vi "Main.vi"(11 "Module Admin":refnum<class "Delacor_lib_QMH_Module Admin.lvclass">) -> ()   [LabVIEW 2024, in "Settings Editor.lvlib"]
doc: "This template is based off of the Queued Message Handler design pattern and the Queued Message Handler project template that ships with LabVIEW.\n\nThe main difference is that the queue is private to this module and communication between modules is performed via Broadcast and Request events.\n\nRequest events are wrapped in public API methods and are handled in the Event Handling Loop (EHL) of this VI. Any module can register for Broadcast events sent by this module. The EHL generates messages based on user interface actions.\n\nThe Message Handling Loop (MHL) processes messages generated by the EHL, or by other messages. The messages are string values, so new messages can be added easily to the Message Cases case structure in the MHL. Each message cluster can also provide an optional value for Message Data, which is a variant that can be converted to whatever message-specific data is required.\n_____\nBased on DQMH Project Template 4.0.0.47.\n_____\nBased on DQMH Dev Tools: Project Template 7.1.0.1503."
uses:
  Settings Editor.lvlib
  <vilib>/Delacor/Delacor QMH/Libraries/Module Admin_class/Delacor_lib_QMH_Module Admin.lvclass
  CML Shared/Signal Type--enum.ctl
  CML Shared/Calibration Values--cluster.ctl
  Module Data--cluster.ctl
  Settings--cluster.ctl
  <vilib>/Delacor/Delacor QMH/Libraries/Message Queue_class/Delacor_lib_QMH_Message Queue.lvclass/Delacor_lib_QMH_Message Queue.ctl
  Stop Argument--cluster.ctl
  Update Application Settings Argument--cluster.ctl
  Update Application Settings (Reply Payload)--cluster.ctl
  <vilib>/Delacor/Delacor QMH/Libraries/Module Admin_class/Delacor_lib_QMH_Module Admin.lvclass/Delacor_lib_QMH_Module Admin.ctl
  <vilib>/Utility/miscctls.llb/LVPointTypeDef.ctl
  <vilib>/Delacor/Delacor QMH/Libraries/Message Queue_class/Delacor_lib_QMH_Enqueue Message (Single).vi
  <vilib>/Delacor/Delacor QMH/Libraries/Module Admin_class/Delacor_lib_QMH_Get External Launch.vi
  <vilib>/Delacor/Delacor QMH/Libraries/Message Queue_class/Delacor_lib_QMH_Message Queue.lvclass
  CML Shared/CML Shared.lvlib
panel:
  in  "Open API TESTERS Window for Debug":bool
  in  "Calibration Values":T1[](array[typedef])
  in  "Cancel":bool
  in  "OK":bool
  in  "Log File Base Path":path
  in  "Signal Type":T2
  out "error out":errorcluster
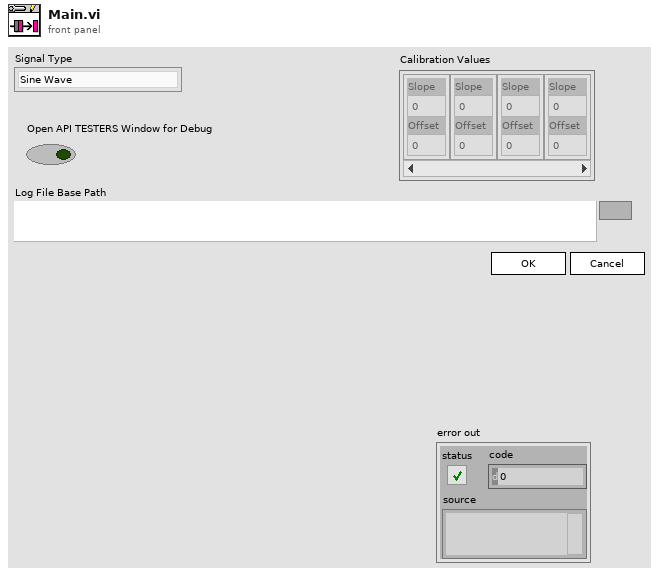
[diagram p1: front panel]
types:
  T1 = typedef "CML Shared.lvlib/Calibration Values--cluster.ctl" = cluster{"Slope":dbl, "Offset":dbl}
  T2 = typedef "CML Shared.lvlib/Signal Type--enum.ctl" = enum16{"Sine Wave", "Square with Noise"}
  T3 = typedef "Settings Editor.lvlib/Request Events--cluster.ctl" = cluster{"Stop Module":refnum<user-event>, "Show Panel":refnum<user-event>, "Hide Panel":refnum<user-event>, "Get Module Execution Status":refnum<user-event>, "Show Diagram":refnum<user-event>, "Update Application Settings":refnum<user-event>}
  T4 = typedef "Settings Editor.lvlib/Module Data--cluster.ctl" = cluster{"Settings":T5}
  T5 = typedef "Settings Editor.lvlib/Settings--cluster.ctl" = cluster{"Signal Type":T2, "Calibration Array":T1[], "Log File Base Path":path}
  T6 = enum32{"invalid lock state", "Not Locked", "Locked (No Password)", "Password-protected"}
  T7 = typedef "Settings Editor.lvlib/Stop Argument--cluster.ctl" = cluster{"Origin":string, "Exit via Stop Module Req?":bool, "Wait for Module to stop?":bool}
  T8 = typedef "Settings Editor.lvlib/Update Application Settings Argument--cluster.ctl" = cluster{"Wait Notifier":refnum<notifier>, "wait for reply":bool}
  T9 = typedef "LVPointTypeDef.ctl" = cluster{"Horizontal":i16, "Vertical":i16}
  T10 = enum32{"Invalid", "Standard", "Closed", "Hidden", "Minimized", "Maximized"}
  T11 = typedef "Settings Editor.lvlib/Update Application Settings (Reply Payload)--cluster.ctl" = cluster{"Settings":T5, "error":errorcluster}
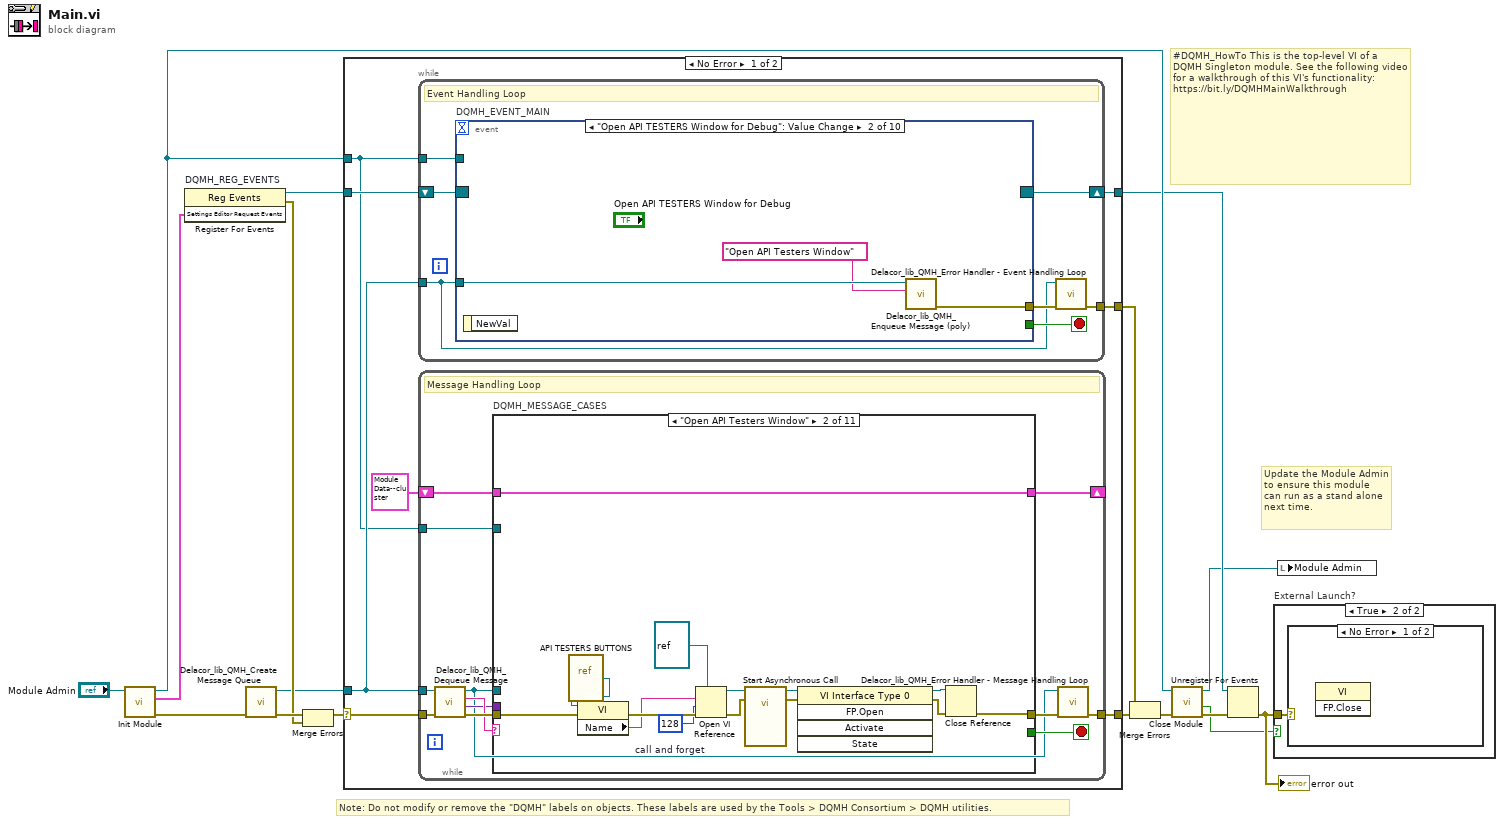
[diagram p0: block diagram]
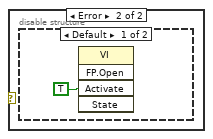
[diagram p3: hidden frame]
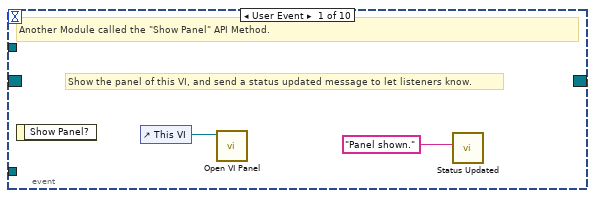
[diagram p5: hidden frame]
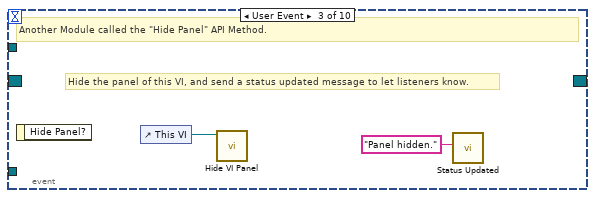
[diagram p6: hidden frame]
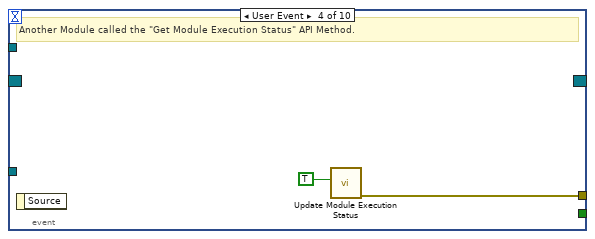
[diagram p7: hidden frame]
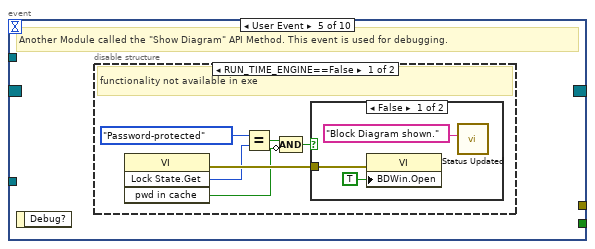
[diagram p8: hidden frame]
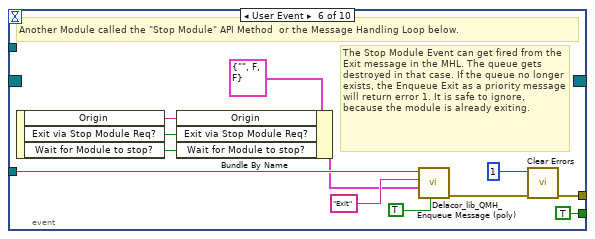
[diagram p11: hidden frame]
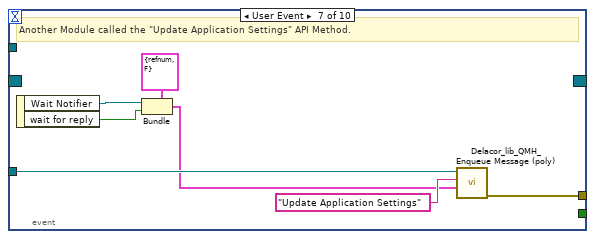
[diagram p12: hidden frame]
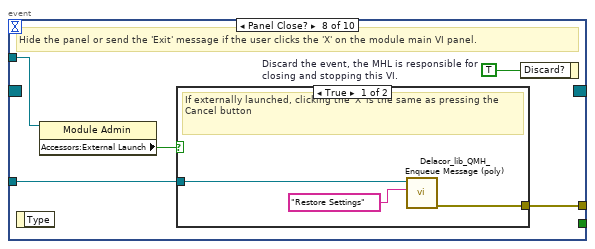
[diagram p13: hidden frame]
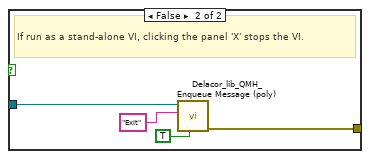
[diagram p14: hidden frame]
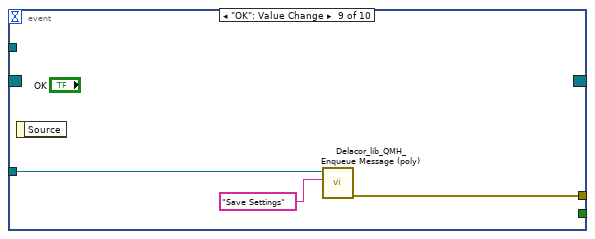
[diagram p15: hidden frame]
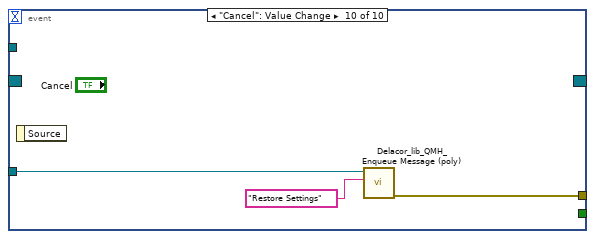
[diagram p16: hidden frame]
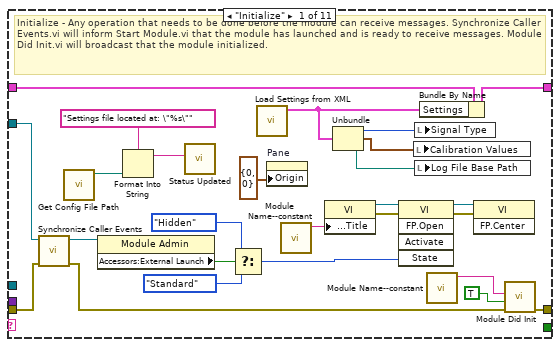
[diagram p17: hidden frame]
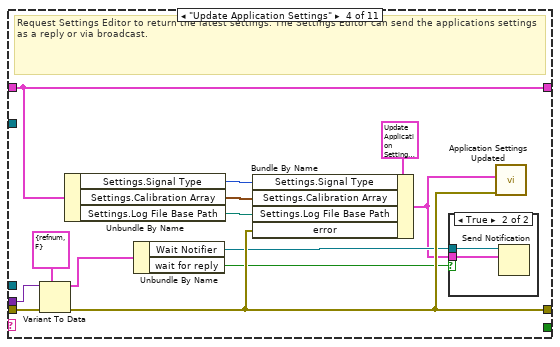
[diagram p19: hidden frame]
diagram:
  # "#DQMH_HowTo This is the top-level VI of a DQMH Singleton module. See the following video for a walkthrough of this VI's functionality: https://bit.ly/DQMHMainWalkthrough"
  # "Note: Do not modify or remove the \"DQMH\" labels on objects. These labels are used by the Tools > DQMH Consortium > DQMH utilities."
  # "Update the Module Admin to ensure this module can run as a stand alone next time."
  n1 = call "Init Module.vi"("Singleton Module Admin in"="Module Admin") -> ("error out"=w16:errorcluster, "Settings Editor Request Events"=w5:T3, "Singleton Module Admin out"=w8:refnum<class "Delacor_lib_QMH_Module Admin.lvclass">)  [unwired: 8 in]
  n2 = register-events "DQMH_REG_EVENTS"(w5) -> (reference out=w6:refnum<event-registration>, error out=w9:errorcluster)  [unwired: 2 in]
  n3 = call <vilib>:"Delacor_lib_QMH_Create Message Queue.vi"("error in"=w16) -> ("error out"=w11:errorcluster, "Message Queue"=w4:refnum<class "Delacor_lib_QMH_Message Queue.lvclass">)  [unwired: 9 in]
  n4 = Merge Errors(w11, w9) -> (w10:errorcluster)
  n5 = case shown="No Error" w10 {
    selector: w10 -> [w23 w230]
    tunnel: [w25 w229] -> w17
    tunnel: [w22 w228] -> w7
    tunnel: w6 -> [w20 w228]
    tunnel: w4 -> [w19 w223]
    tunnel: [w24 _] -> w14
    tunnel: w8 -> [w18 w224]
    frame No Error {
      n6 = while {
        tunnel: w19 -> [w26]
        shift-right: [w29] -> w22
        shift-left: w20 -> [w30]
        tunnel: [w31] -> w24
        tunnel: w18 -> [w27]
        stop <- w28 stop-if-true
        # "Event Handling Loop"
        n7 = event "DQMH_EVENT_MAIN" shown="[1] \"Open API TESTERS Window for Debug\": Value Change" {
          selector: w30 -> [_ _ _ _ _ _ _ _ _ _]
          dyn-events: [_ _ _ _ _ _ _ _ _ _] -> w29
          timeout: _ -> [_ _ _ _ _ _ _ _ _ _]
          tunnel: [_ _ _ _ _ TRUE ("Discard?") _ _ _ _] -> w28
          tunnel: w26 -> [_ w36 _ _ _ w58 w68 w72 w82 w85]
          tunnel: [_ w37 _ w41 _ w61 w69 w74 w84 w87] -> w32
          tunnel: w27 -> [_ _ _ _ _ _ _ w71 _ _]
          event User Event {
            # "Show the panel of this VI, and send a status updated message to let listeners know."
            # "Another Module called the \"Show Panel\" API Method."
            n8 = event-data() -> ()  [unwired: 1 in, 1 out]
            n9 = control-ref of="This VI"() -> (w34:refnum<vi>)
            n10 = call "Open VI Panel.vi"("VI"=w34) -> ()  [unwired: 10 in, 1 out]
            n11 = call "Status Updated.vi"("Status"="Panel shown." ("format string")) -> ()  [unwired: 10 in, 1 out]
          }
          event "Open API TESTERS Window for Debug": Value Change {
            n12 = event-data() -> ()  [unwired: 1 in, 1 out]
            n13 = call-poly <vilib>:"Delacor_lib_QMH_Enqueue Message (poly).vi"("Message"="Open API Testers Window", "Message Queue in"=w36) -> ("error out"=w37:errorcluster)  [unwired: 8 in, 1 out]
          }
          event User Event {
            # "Hide the panel of this VI, and send a status updated message to let listeners know."
            # "Another Module called the \"Hide Panel\" API Method."
            n14 = event-data() -> ()  [unwired: 1 in, 1 out]
            n15 = control-ref of="This VI"() -> (w39:refnum<vi>)
            n16 = call "Hide VI Panel.vi"("VI"=w39) -> ()  [unwired: 10 in, 1 out]
            n17 = call "Status Updated.vi"("Status"="Panel hidden." ("format string")) -> ()  [unwired: 10 in, 1 out]
          }
          event User Event {
            # "Another Module called the \"Get Module Execution Status\" API Method."
            n18 = event-data() -> ()  [unwired: 1 in, 1 out]
            n19 = call "Update Module Execution Status.vi"("Running?"=TRUE) -> ("error out"=w41:errorcluster)  [unwired: 10 in]
          }
          event User Event {
            # "Another Module called the \"Show Diagram\" API Method. This event is used for debugging."
            n20 = event-data() -> ()  [unwired: 1 in, 1 out]
            n21 = disable-structure shown="RUN_TIME_ENGINE==False" {
              frame condition #0 (active) {
                # "functionality not available in exe"
                n22 = invoke on="Invoke Node" class="VI" method="Lock State.Get"() -> (error out=w47:errorcluster, "Get Lock State"=w46:T6, "pwd in cache"=w43:bool)  [unwired: 4 in, 1 out]
                n23 = Equal?(x=T6."Password-protected", y=w46) -> (x = y?=w44:bool)
                n24 = Compound Arithmetic op=AND(w44, invert w43) -> (w42:bool)
                n25 = case shown="False" w42 {
                  tunnel: w47 -> [w50 _]
                  frame False {
                    n26 = property on="Property Node" class="VI"(error in=w50, "BDWin.Open"=TRUE ("Block Diagram Window:Open")) -> ()  [unwired: 1 in, 2 out]
                    n27 = call "Status Updated.vi"("Status"="Block Diagram shown." ("format string")) -> ()  [unwired: 10 in, 1 out]
                  }
                  frame True {
                    # "Password-protected VI, and the password is not in the cache. Do not show the diagram."
                  }
                }
              }
              frame condition #1 {
              }
            }
          }
          event User Event {
            # "The Stop Module Event can get fired from the Exit message in the MHL. The queue gets destroyed in that case. If the queue no longer exists, the Enqueue Exit as a priority message will return error 1. It is safe to ignore, because the module is already exiting."
            # "Another Module called the \"Stop Module\" API Method  or the Message Handling Loop below."
            n28 = event-data() -> ("Origin"=w51:string, "Exit via Stop Module Req?"=w54:bool, "Wait for Module to stop?"=w53:bool)  [unwired: 1 in]
            n29 = Bundle By Name(cluster=T7 {"Origin"="", "Exit via Stop Module Req?"=FALSE, "Wait for Module to stop?"=FALSE} ("Stop Argument"), "Origin"=w51, "Exit via Stop Module Req?"=w54, "Wait for Module to stop?"=w53) -> (w52:T7)
            n30 = call-poly <vilib>:"Delacor_lib_QMH_Enqueue Message (poly).vi"("Priority Message? (F)"=TRUE, "Message Data"=w52, "Message"="Exit", "Message Queue in"=w58) -> ("error out"=w62:errorcluster)  [unwired: 6 in, 1 out]
            n31 = call <vilib>:"Clear Errors.vi"("error in (no error)"=w62, "specific error code to clear (0: all)"=1) -> ("error out"=w61:errorcluster)  [unwired: 4 in, 1 out]
          }
          event User Event {
            # "Another Module called the \"Update Application Settings\" API Method."
            n32 = event-data() -> ("Wait Notifier"=w64:refnum<notifier>, "wait for reply"=w63:bool)  [unwired: 1 in]
            n33 = Bundle(cluster=T8 {"Wait Notifier"=refnum, "wait for reply"=FALSE} ("Update Application Settings Argument"), "Wait Notifier"=w64, "wait for reply"=w63) -> (w65:T8)
            n34 = call-poly <vilib>:"Delacor_lib_QMH_Enqueue Message (poly).vi"("Message Data"=w65, "Message"="Update Application Settings", "Message Queue in"=w68) -> ("error out"=w69:errorcluster)  [unwired: 7 in, 1 out]
          }
          event Panel Close? {
            w73 = TRUE  # Discard the event, the MHL is responsible for closing and stopping this VI.
            # "Hide the panel or send the 'Exit' message if the user clicks the 'X' on the module main VI panel."
            n35 = event-data() -> ()  [unwired: 1 in, 1 out]
            n36 = property on="Property Node" class="Module Admin"(reference=w71) -> ("Accessors:External Launch"=w70:bool)  [unwired: 1 in, 2 out]
            n37 = case shown="True" w70 {
              tunnel: w72 -> [w75 w80]
              tunnel: [w77 w81] -> w74
              frame True {
                # "If externally launched, clicking the 'X' is the same as pressing the Cancel button"
                n38 = call-poly <vilib>:"Delacor_lib_QMH_Enqueue Message (poly).vi"("Message"="Restore Settings", "Message Queue in"=w75) -> ("error out"=w77:errorcluster)  [unwired: 8 in, 1 out]
              }
              frame False {
                # "If run as a stand-alone VI, clicking the panel 'X' stops the VI."
                n39 = call-poly <vilib>:"Delacor_lib_QMH_Enqueue Message (poly).vi"("Priority Message? (F)"=TRUE, "Message"="Exit", "Message Queue in"=w80) -> ("error out"=w81:errorcluster)  [unwired: 7 in, 1 out]
              }
            }
            n40 = event-data ("Event Filter Node")("Discard?"=w73) -> ()  [unwired: 1 in, 1 out]
          }
          event "OK": Value Change {
            n41 = event-data() -> ()  [unwired: 1 in, 1 out]
            n42 = call-poly <vilib>:"Delacor_lib_QMH_Enqueue Message (poly).vi"("Message"="Save Settings", "Message Queue in"=w82) -> ("error out"=w84:errorcluster)  [unwired: 8 in, 1 out]
          }
          event "Cancel": Value Change {
            n43 = event-data() -> ()  [unwired: 1 in, 1 out]
            n44 = call-poly <vilib>:"Delacor_lib_QMH_Enqueue Message (poly).vi"("Message"="Restore Settings", "Message Queue in"=w85) -> ("error out"=w87:errorcluster)  [unwired: 8 in, 1 out]
          }
        }
        n45 = call-dynamic "Delacor_lib_QMH_Error Handler - Event Handling Loop.vi"("error in"=w32, "Message Queue in"=w26) -> ("dup error in"=w31:errorcluster)  [unwired: 8 in, 1 out]
      }
      n46 = while {
        tunnel: w19 -> [w90]
        shift-right: [w94] -> _
        shift-left: T4 {"Settings"={"Signal Type"=enum."Sine Wave", "Calibration Array"=[{"Slope"=1.0, "Offset"=0.0}], "Log File Base Path"=path ""}} ("Data Cluster") -> [w95]
        tunnel: w23 -> [w98]
        tunnel: [w96] -> w25
        tunnel: w18 -> [w88]
        stop <- w93 stop-if-true
        # "Message Handling Loop"
        n47 = call-dynamic "Delacor_lib_QMH_Dequeue Message.vi"("error in"=w98, "Message Queue in"=w90) -> ("error out"=w97:errorcluster, "Message Data"=w91:variant, "Message"=w92:string, "Message Queue out"=w89:refnum<class "Delacor_lib_QMH_Message Queue.lvclass">)  [unwired: 6 in]
        n48 = case "DQMH_MESSAGE_CASES" shown="\"Open API Testers Window\"" w92 {
          selector: w92 -> [_ _ _ _ _ _ _ _ _ _ w218]
          tunnel: w89 -> [_ _ _ _ _ _ _ _ w184 w206 _]
          tunnel: w97 -> [w124 w128 w141 w153 w168 w175 w178 w180 w191 w212 w221]
          tunnel: [w122 w126 w141 w154 w169 w175 w177 w180 w187 w207 w222] -> w99
          tunnel: w95 -> [w112 w139 w140 w147 w165 w174 w176 w179 w186 w205 w219]
          tunnel: [w111 w139 w140 w147 w162 w174 w176 w179 w186 w205 w219] -> w94
          tunnel: [_ _ _ _ _ _ _ _ _ w204 _] -> w93
          tunnel: w91 -> [_ _ _ w152 _ _ _ _ w185 w203 _]
          tunnel: w88 -> [w113 _ _ _ _ _ _ _ w183 w198 _]
          frame "Initialize" {
            # "Initialize - Any operation that needs to be done before the module can receive messages. Synchronize Caller Events.vi will inform Start Module.vi that the module has launched and is ready to receive messages. Module Did Init.vi will broadcast that the module initialized."
            n49 = call "Synchronize Caller Events.vi"("error in"=w124, "Singleton Module Admin in"=w113) -> ("error out"=w123:errorcluster, "Singleton Module Admin out"=w108:refnum<class "Delacor_lib_QMH_Module Admin.lvclass">)  [unwired: 8 in]
            n50 = call "Get Config File Path.vi"() -> ("XML File Path"=w106:path)  [unwired: 10 in, 1 out]
            n51 = property on="Property Node" class="Module Admin"(reference=w108) -> ("Accessors:External Launch"=w117:bool)  [unwired: 1 in, 2 out]
            n52 = Format Into String(format string="Settings file located at: \"%s\"", w106) -> (resulting string=w105:string)  [unwired: 2 in, 1 out]
            n53 = call "Status Updated.vi"("Status"=w105) -> ()  [unwired: 10 in, 1 out]
            n54 = Select(t=T10."Hidden" ("State"), s=w117, f=T10."Standard" ("State")) -> (s? t:f=w114:T10)
            n55 = call "Load Settings from XML.vi"() -> ("Settings out"=w103:T5)  [unwired: 10 in, 1 out]
            n56 = property on="Pane" class="Pane"("Origin"=T9 {"Horizontal"=0, "Vertical"=0}) -> ()  [unwired: 2 in, 2 out]
            n57 = call "Module Name--constant.vi"() -> ("Module Name"=w120:string)  [unwired: 11 in]
            n58 = property on="Property Node" class="VI"("Front Panel.Title"=w120) -> (reference out=w119:refnum<vi>, error out=w121:errorcluster)  [unwired: 2 in]
            n59 = Unbundle(w103) -> ("Signal Type"=w102:T2, "Calibration Array"=w101:T1[], "Log File Base Path"=w100:path)
            n60 = invoke on="Invoke Node" class="VI" method="FP.Open"(reference=w119, error in=w121, "State"=w114) -> (reference out=w118:refnum<vi>, error out=w125:errorcluster)  [unwired: 2 in, 3 out]
            n61 = local write "Calibration Values"(w101) -> ()
            n62 = local write "Signal Type"(w102) -> ()
            n63 = local write "Log File Base Path"(w100) -> ()
            n64 = Bundle By Name(cluster=w112, "Settings"=w103) -> (w111:T4)
            n65 = call "Module Name--constant.vi"() -> ("Module Name"=w109:string)  [unwired: 11 in]
            n66 = invoke on="Invoke Node" class="VI" method="FP.Center"(reference=w118, error in=w125) -> ()  [unwired: 1 in, 3 out]
            n67 = call "Module Did Init.vi"("error in"=w123, "Initialized?"=TRUE, "Origin"=w109) -> ("error out"=w122:errorcluster)  [unwired: 8 in]
          }
          frame "Open API Testers Window" {
            w129 = 128  # call and forget
            n68 = vi-ref "API TESTERS BUTTONS.vi"() -> (w127:refnum<vi>)
            n69 = property class="VI"(reference=w127, error in=w128) -> (error out=w138:errorcluster, "Name"=w134:string)  [unwired: 1 out]
            n70 = Open VI Reference(type specifier VI Refnum (for type only)=refnum<vi> refnum, vi path=w134, options=w129, error in (no error)=w138) -> (vi reference=w132:refnum<vi>, error out=w137:errorcluster)  [unwired: 2 in]
            n71 = call-by-ref "Start Asynchronous Call"(reference=w132, error in=w137) -> (reference out=w131:refnum<vi>, error out=w136:errorcluster)  [unwired: 12 in]
            n72 = invoke class="VI Interface Type 0" method="FP.Open"(reference=w131, error in=w136) -> (reference out=w130:refnum<vi>, error out=w135:errorcluster)  [unwired: 3 in, 3 out]
            n73 = Close Reference(reference=w130, error in (no error)=w135) -> (error out=w126:errorcluster)
          }
          frame "---Module Specific---" {
            # "Separator -- The following cases handle messages specific to this Module."
          }
          frame "Update Application Settings" {
            # "Request Settings Editor to return the latest settings. The Settings Editor can send the applications settings as a reply or via broadcast."
            n74 = Variant To Data(error in=w153, type=T8 {"Wait Notifier"=refnum, "wait for reply"=FALSE} ("Update Application Settings Argument"), Variant=w152) -> (data=w150:T8, error out=w154:errorcluster)
            n75 = Unbundle By Name(w147) -> ("Settings.Signal Type"=w145:T2, "Settings.Calibration Array"=w144:T1[], "Settings.Log File Base Path"=w143:path)
            n76 = Unbundle By Name(w150) -> ("Wait Notifier"=w149:refnum<notifier>, "wait for reply"=w148:bool)
            n77 = Bundle By Name(cluster=T11 {"Settings"={"Signal Type"=enum."Sine Wave", "Calibration Array"=[], "Log File Base Path"=path ""}, "error"={"status"=FALSE, "code"=0, "source"=""}} ("Update Application Settings (Reply Payload)"), "Settings.Signal Type"=w145, "Settings.Calibration Array"=w144, "Settings.Log File Base Path"=w143, "error"=w154) -> (w142:T11)
            n78 = case shown="True" w148 {
              tunnel: w149 -> [_ w156]
              tunnel: w142 -> [_ w155]
              frame False {
              }
              frame True {
                n79 = Send Notification(notification=w155, notifier=w156) -> ()  [unwired: 1 in, 2 out]
              }
            }
            n80 = call "Application Settings Updated.vi"("error in"=w154, "Reply Payload"=w142) -> ()  [unwired: 9 in, 1 out]
          }
          frame "Save Settings" {
            # "The end user pressed OK button and the current values on the front panel are the new settings."
            n81 = Bundle By Name(cluster=w165, "Settings.Calibration Array"="Calibration Values", "Settings.Signal Type"="Signal Type", "Settings.Log File Base Path"="Log File Base Path") -> (w162:T4)
            n82 = Unbundle By Name(w162) -> ("Settings"=w157:T5)
            n83 = Bundle By Name(cluster=T11 {"Settings"={"Signal Type"=enum."Sine Wave", "Calibration Array"=[], "Log File Base Path"=path ""}, "error"={"status"=FALSE, "code"=0, "source"=""}} ("Reply Payload"), "Settings"=w157) -> (w158:T11)
            n84 = control-ref of="This VI"() -> (w163:refnum<vi>)
            n85 = call "Application Settings Updated.vi"("Reply Payload"=w158) -> ("error out"=w166:errorcluster)  [unwired: 10 in]
            n86 = call "Save Settings to XML.vi"("Settings"=w157) -> ("error out"=w167:errorcluster)  [unwired: 10 in]
            n87 = call "Hide VI Panel.vi"("VI"=w163) -> ()  [unwired: 10 in, 1 out]
            n88 = Merge Errors(w168, w167, w166) -> (w169:errorcluster)
          }
          frame "Restore Settings" {
            # "The end user pressed Cancel button, need to restore the current stored values for the controls on the front panel. No need to broadcast that the settings changed."
            n89 = Unbundle By Name(w174) -> ("Settings.Signal Type"=w173:T2, "Settings.Log File Base Path"=w172:path)
            n90 = control-ref of="This VI"() -> (w171:refnum<vi>)
            n91 = call "Hide VI Panel.vi"("VI"=w171) -> ()  [unwired: 10 in, 1 out]
            n92 = local write "Signal Type"(w173) -> ()
            n93 = local write "Log File Base Path"(w172) -> ()
            n94 = call "Status Updated.vi"("Status"="Panel hidden." ("format string")) -> ()  [unwired: 10 in, 1 out]
          }
          frame "---Copy This Frame---" {
            # "Duplicate this frame when creating new messages.  Change this comment in the duplicated frame to describe this message."
            n95 = Merge Errors(w178) -> (w177:errorcluster)
          }
          frame "---Exit and Error Handling---" {
            # "Separator - The following cases handle errors and exit messages."
          }
          frame "Error" {
            # "Error - Check the error message data and respond accordingly. This message is sent by the \"Error Handler\" VIs at the end of each loop in this application."
            n96 = property on="Property Node" class="Module Admin"(reference=w183) -> ("Accessors:External Launch"=w182:bool)  [unwired: 1 in, 2 out]
            n97 = Variant To Data(error in=w191, type=errorcluster {"status"=FALSE, "code"=0, "source"=""} ("error constant"), Variant=w185) -> (data=w181:errorcluster, error out=w189:errorcluster)
            n98 = local write "error out"(w181) -> ()
            n99 = call "Error Reported.vi"("Error"=w181) -> ()  [unwired: 10 in, 1 out]
            n100 = case shown="False" w182 {
              tunnel: [w196 _] -> w188
              tunnel: w184 -> [w194 _]
              tunnel: w181 -> [w195 _]
              frame False {
                n101 = disable-structure shown="Default" {
                  disable-tunnel: w195 -> [w197 _]
                  frame condition #0 (active) {
                    # "If the module is running standalone, then pop up an error dialog and call the \"Exit\" message."
                    n102 = call <vilib>:"Simple Error Handler.vi"("error in (no error)"=w197) -> ()  [unwired: 4 in, 5 out]
                  }
                  frame condition #1 {
                    # "To prevent the Simple Error Handler VI from being loaded (e.g. when deploying to a Real-Time target), add the Conditional Disable Symbol \"DQMH_Disable_SEH\" to your project and set it to TRUE."
                  }
                }
                n103 = call-poly <vilib>:"Delacor_lib_QMH_Enqueue Message (poly).vi"("Priority Message? (F)"=TRUE, "Message"="Exit", "Message Queue in"=w194) -> ("error out"=w196:errorcluster)  [unwired: 7 in, 1 out]
              }
              frame True {
                # "If the module was launched externally, calling the Error Reported broadcast VI is the only action performed by the \"Error\" message. The module's caller can then process the error appropriately."
              }
            }
            n104 = Merge Errors(w189, w188) -> (w187:errorcluster)
          }
          frame "Exit" {
            w204 = TRUE  # Stop the VI
            # "Release the message queue reference"
            # "Exit - Exit the application."
            n105 = Variant To Data(error in=w212, type=T7 {"Origin"="", "Exit via Stop Module Req?"=FALSE, "Wait for Module to stop?"=FALSE} ("Stop Argument"), Variant=w203) -> (data=w200:T7, error out=w209:errorcluster)
            n106 = call <vilib>:"Clear Errors.vi"("error in (no error)"=w209, "specific error code to clear (0: all)"=91 ("91: not all Exit messages will have an argument")) -> ("error out"=w211:errorcluster)  [unwired: 4 in, 1 out]
            n107 = control-ref of="This VI"() -> (w199:refnum<vi>)
            n108 = call-dynamic "Delacor_lib_QMH_Release Message Queue.vi"("error in"=w211, "Message Queue"=w206) -> ("error out"=w210:errorcluster)  [unwired: 9 in]
            n109 = call "Handle Exit.vi"("Stop Argument"=w200, "Admin in"=w198, "VI reference"=w199) -> ("error out"=w208:errorcluster)  [unwired: 7 in, 1 out]
            n110 = Merge Errors(w210, w208) -> (w207:errorcluster)
            n111 = call "Error Reported.vi"("Error"=w207) -> ()  [unwired: 10 in, 1 out]
          }
          frame Default {
            # "'Default' case only runs if there is a message that isn't defined in any of the other cases.  Output a programming error."
            n112 = call "Module Name--constant.vi"() -> ("Module Name"=w217:string)  [unwired: 11 in]
            n113 = Format Into String(format string="The invalid message string \"%s\" was received in the Message Handling Loop for module \"%s\".", w218, w217) -> (resulting string=w215:string)  [unwired: 2 in, 1 out]
            n114 = call <vilib>:"Error Cluster From Error Code.vi"("show call chain? (False)"=TRUE, "error message (\"\")"=w215, "error code (0)"=1) -> ("error out"=w220:errorcluster)  [unwired: 6 in]
            n115 = Merge Errors(w221, w220) -> (w222:errorcluster)
          }
        }
        n116 = call-dynamic "Delacor_lib_QMH_Error Handler - Message Handling Loop.vi"("error in"=w99, "Message Queue in"=w89) -> ("dup error in"=w96:errorcluster)  [unwired: 8 in, 1 out]
      }
    }
    frame Error {
      # "Synchronize Caller Events.vi will inform Start Module.vi that the module has launched and will let the code calling Start Module.vi register for broadcasts and would permit the caller receive the broadcast that an error occurred at launch time."
      n117 = call "Synchronize Caller Events.vi"("Singleton Module Admin in"=w224) -> ("error out"=w231:errorcluster)  [unwired: 9 in, 1 out]
      n118 = call-dynamic "Delacor_lib_QMH_Release Message Queue.vi"("error in"=w230, "Message Queue"=w223) -> ("error out"=w229:errorcluster)  [unwired: 9 in]
      n119 = call "Module Name--constant.vi"() -> ("Module Name"=w227:string)  [unwired: 11 in]
      n120 = Format Into String(format string="An error occurred during initialization. %s is no longer running.", w227) -> (resulting string=w225:string)  [unwired: 2 in, 1 out]
      n121 = Merge Errors(w229, w231) -> (w232:errorcluster)
      n122 = call "Error Reported.vi"("Additional Information"=w225, "Error"=w232) -> ()  [unwired: 9 in, 1 out]
    }
  }
  n123 = Merge Errors(w14, w17) -> (w13:errorcluster)
  n124 = call "Close Module.vi"("error in"=w13, "Module Admin in"=w8) -> ("error out"=w15:errorcluster, "External Launch"=w1:bool, "Module Admin out"=w2:refnum<class "Delacor_lib_QMH_Module Admin.lvclass">)  [unwired: 7 in]
  n125 = Unregister For Events(event registration refnum=w7, error in=w15) -> (error out=w12:errorcluster)
  "error out" <- w12
  n126 = case "External Launch?" shown="True" w1 {
    tunnel: w12 -> [_ w233]
    frame False {
    }
    frame True {
      n127 = case shown="No Error" w233 {
        frame No Error {
          n128 = invoke on="Invoke Node" class="VI" method="FP.Close"() -> ()  [unwired: 3 in, 3 out]
        }
        frame Error {
          n129 = disable-structure shown="Default" {
            frame condition #0 (active) {
              n130 = invoke class="VI" method="FP.Open"("Activate"=TRUE ("Activate?")) -> ()  [unwired: 4 in, 5 out]
            }
            frame condition #1 {
              # "Don't show panel on error if running inside a built EXE."
            }
          }
        }
      }
    }
  }
  n131 = local write "Module Admin"(w2) -> ()
